vi "Find Row Reflection of 2D array.vi"(11 "2D array":bool[][](array[boolean])) -> (2 "Reflection found":bool, 3 "Row index of reflection":i32)   [LabVIEW 2023]
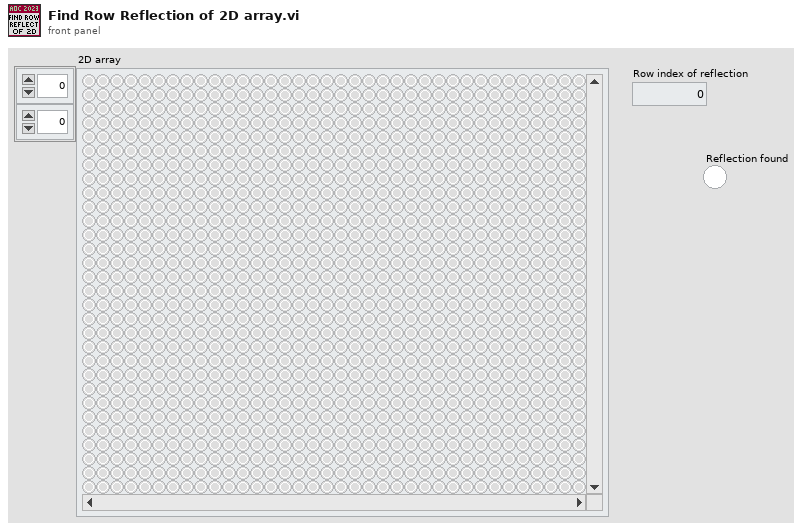
[diagram p1: front panel]
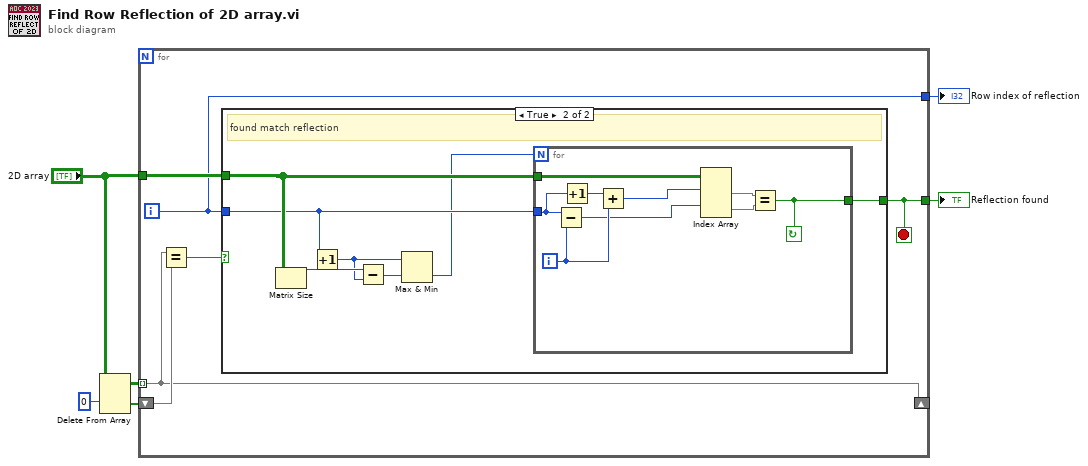
[diagram p0: block diagram]
diagram:
  n1 = Delete From Array(array="2D array", index (row)=0) -> (deleted portion=w2:bool[], array with subset deleted=w3:bool[][])  [unwired: 2 in]
  n2 = for {
    shift-right: [w11] -> _
    shift-left: w2 -> [w12]
    tunnel: w3 -> [w11] mode=indexing
    tunnel: "2D array" -> [w9]
    tunnel: [w8] -> w5
    tunnel: [w7] -> w6
    i -> [w7]
    stop <- w8 stop-if-true
    n3 = Equal?(x=w11, y=w12) -> (x = y?=w10:bool)
    n4 = case shown="True" w10 {
      selector: w10 -> [w13 _]
      tunnel: w9 -> [_ w19]
      tunnel: w7 -> [_ w17]
      tunnel: [w13 w20] -> w8
      frame False {
        # "Ajacent rows do not match"
      }
      frame True {
        # "found match reflection"
        n5 = Matrix Size(0:w19) -> (1:w18:i32)  [unwired: 1 out]
        n6 = Increment(x=w17) -> (x+1=w15:i32)
        n7 = Subtract(x=w18, y=w15) -> (x-y=w16:i32)
        n8 = Max & Min(x=w15, y=w16) -> (min(x,y)=w14:i32)  [unwired: 1 out]
        n9 = for {
          N: w14 -> [_]
          tunnel: w19 -> [w26]
          tunnel: w17 -> [w29]
          tunnel: [w21] -> w20
          i -> [w27]
          stop <- w21 continue-if-true
          n10 = Subtract(x=w29, y=w27) -> (x-y=w24:i32)
          n11 = Increment(x=w29) -> (x+1=w28:i32)
          n12 = Add(x=w28, y=w27) -> (x+y=w25:i32)
          n13 = Index Array(array=w26, index (row) #1=w25, index (row) #2=w24) -> (element #1=w23:bool[], element #2=w22:bool[])  [unwired: 2 in]
          n14 = Equal?(x=w23, y=w22) -> (x = y?=w21:bool)
        }
      }
    }
  }
  "Row index of reflection" <- w6
  "Reflection found" <- w5
